vi "Window_Assignment.vi"(8 "error in (no error)":errorcluster, 9 "stop":bool, 10 "Iteration":i32, 11 "FrameRate":dbl) -> (2 "Stop Sample":bool, 3 "Window Number":i64)   [LabVIEW 2020]
uses:
  Global Variables/Window_Size.vi
  Global Variables/Number_of_Windows.vi
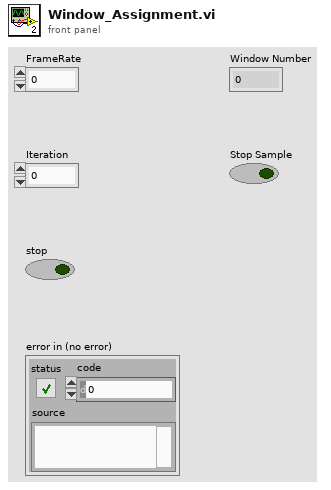
[diagram p1: front panel]
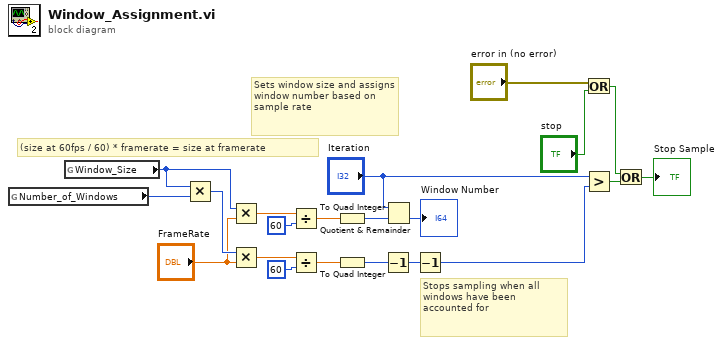
[diagram p0: block diagram]
diagram:
  # "(size at 60fps / 60) * framerate = size at framerate"
  # "Stops sampling when all windows have been accounted for"
  # "Sets window size and assigns window number based on sample rate"
  n1 = global read "Number_of_Windows.vi" "Number_of_Windows"() -> (w1:i64)
  n2 = global read "Window_Size.vi" "Window_Size"() -> (w6:i64)
  n3 = Multiply(x=w6, y=w1) -> (x*y=w7:i64)
  n4 = Multiply(x=w6, y="FrameRate") -> (x*y=w3:dbl)
  n5 = Multiply(x=w7, y="FrameRate") -> (x*y=w8:dbl)
  n6 = Divide(x=w3, y=60) -> (x/y=w2:dbl)
  n7 = Divide(x=w8, y=60) -> (x/y=w14:dbl)
  n8 = To Quad Integer(1:w2) -> (0:w18:i64)
  n9 = To Quad Integer(1:w14) -> (0:w15:i64)
  n10 = Decrement(x=w15) -> (x-1=w16:i64)
  n11 = Quotient & Remainder(x="Iteration", y=w18) -> (floor(x/y)=→"Window Number":i64)  [unwired: 1 out]
  n12 = Decrement(x=w16) -> (x-1=w17:i64)
  n13 = Or(x="error in (no error)", y="stop") -> (x .or. y?=w12:bool)
  n14 = Greater?(x="Iteration", y=w17) -> (0:w11:bool)
  n15 = Or(x=w12, y=w11) -> (x .or. y?=→"Stop Sample":bool)
